vi "PWM Write Frequency.vi"(7 "GPIO #":T1=-1, 8 "error in (no error)":errorcluster, 10 "Frequency Hz":sgl, 11 "Session in":refnum<class "Session.lvclass">) -> (0 "error out":errorcluster, 3 "Session out":refnum<class "Session.lvclass">)   [LabVIEW 2024, in "CTI.lvlib" / "Session.lvclass"]
doc: "Sets the frequency the PWM output will operate at. This is the number of transitions from low to high that happen in a single second. Some peripherals require specific frequency ranges for proper operation while other peripherals can handle a wider range fo frequencies. RC Servos typically operate at 50Hz but controlling brightness of an LED may produce visible flickering unless higher frequencies are specified."
uses:
  Session.lvclass
  GPIO Number.ctl
  DeviceComms/DeviceComms.lvclass
  CTI.lvlib
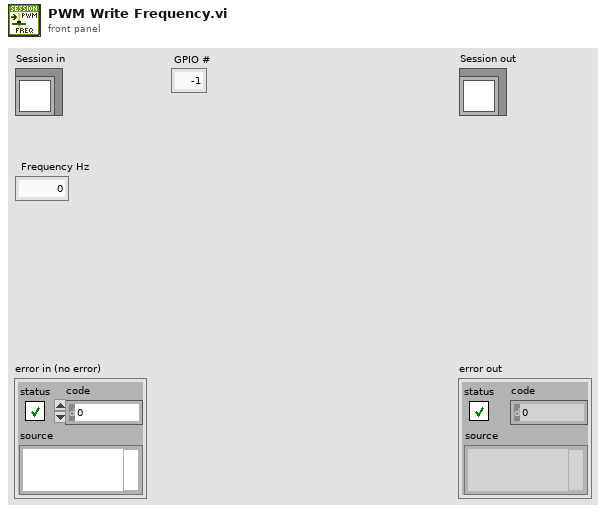
[diagram p1: front panel]
types:
  T1 = typedef "CTI.lvlib/GPIO Number.ctl" = i8
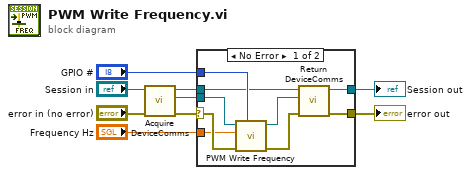
[diagram p0: block diagram]
diagram:
  n1 = call "Acquire DeviceComms.vi"("error in (no error)"="error in (no error)", "Session in"="Session in") -> ("error out"=w8:errorcluster, "DeviceComms"=w7:refnum<class "DeviceComms.lvclass">, "Session out"=w9:refnum<class "Session.lvclass">)  [unwired: 7 in]
  n2 = case shown="No Error" w8 {
    selector: w8 -> [w18 w19]
    tunnel: w9 -> [w14 w20]
    tunnel: w7 -> [w17 _]
    tunnel: "GPIO #" -> [w16 _]
    tunnel: "Frequency Hz" -> [w15 _]
    tunnel: [w11 w19] -> w2
    tunnel: [w10 w20] -> w1
    frame No Error {
      n3 = call-dynamic "PWM Write Frequency.vi"("GPIO #"=w16, "error in (no error)"=w18, "Frequency Hz"=w15, "DeviceComms in"=w17) -> ("error out"=w12:errorcluster, "DeviceComms out"=w13:refnum<class "DeviceComms.lvclass">)  [unwired: 6 in]
      n4 = call "Return DeviceComms.vi"("error in (no error)"=w12, "DeviceComms"=w13, "Session in"=w14) -> ("error out"=w11:errorcluster, "Session out"=w10:refnum<class "Session.lvclass">)  [unwired: 7 in]
    }
    frame Error {
    }
  }
  "error out" <- w2
  "Session out" <- w1
